vi "Pendulum query.vi"(9 "timeout_sec":dbl, 10 "retry_ms":dbl, 11 "instance":i32) -> (3 "function return":i32)   [LabVIEW 2024, in "pendulumApp.lvlib"]
doc: "OOTB_API int Pendulum_query(int instance,double retry_ms, double timeout_sec);"
uses:
  pendulumApp.lvlib
  pendulumApp.dll
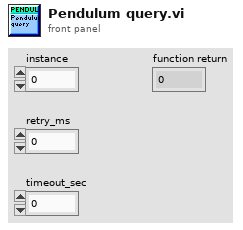
[diagram p1: front panel]
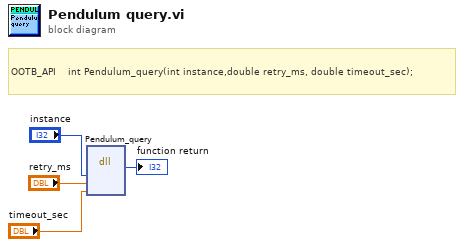
[diagram p0: block diagram]
diagram:
  # "OOTB_API    int Pendulum_query(int instance,double retry_ms, double timeout_sec);"
  n1 = dll-call lib="C:/Users/scer/OneDrive - University of Florida/eml4314c/eml4314cFA25/Resources/FA25_dev_version2/SADI_Pendulum_lib/pendulumApp.*" fn="Pendulum_query"("instance"="instance", "retry_ms"="retry_ms", "timeout_sec"="timeout_sec") -> ("return type"=→"function return":i32)  [unwired: 6 in, 2 out]
